vi "create demo setpoint.vi"(4 "setpoint type":T1(ring)=enum."square", 5 "manual input":dbl format="%.2f") -> (1 "setpoint":dbl(graph), 2 "show slider":bool)   [LabVIEW 2016]
doc: "This subVI creates changing set point values for the PID to track. You can choose from:\n\nsin\nsinc\natan\nsquare\ntriangle\nsawtooth\nrandom\nmanual"
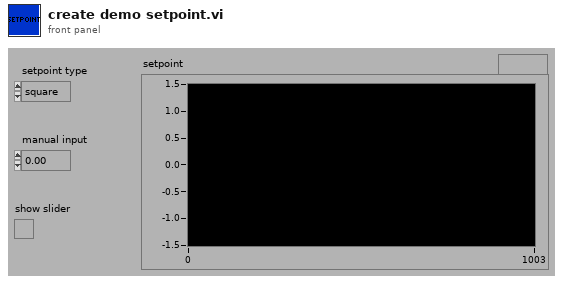
[diagram p1: front panel]
types:
  T1 = enum16{"sine", "sinc", "atan", "square", "triangle", "sawtooth", "random", "manual"}
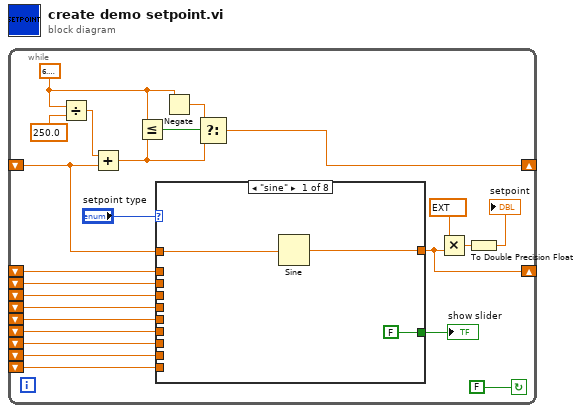
[diagram p0: block diagram]
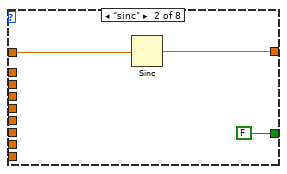
[diagram p2: hidden frame]
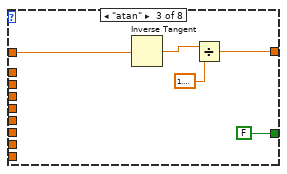
[diagram p3: hidden frame]
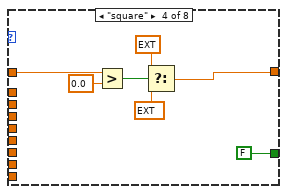
[diagram p4: hidden frame]
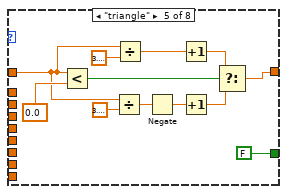
[diagram p5: hidden frame]
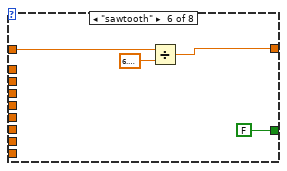
[diagram p6: hidden frame]
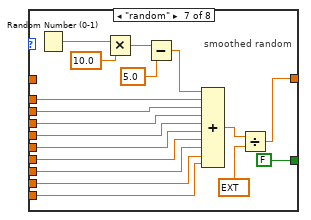
[diagram p7: hidden frame]
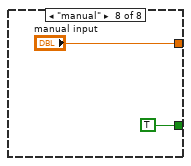
[diagram p8: hidden frame]
diagram:
  n1 = while {
    shift-left: _ -> [w8]
    shift-left: _ -> [w9]
    shift-left: _ -> [w10]
    shift-left: _ -> [w11]
    shift-left: _ -> [w13]
    shift-left: _ -> [w12]
    shift-left: _ -> [w15]
    shift-left: _ -> [w14]
    shift-left: _ -> [w16]
    shift-right: [w4] -> _
    shift-left: _ -> [w18]
    shift-right: [w17] -> _
    stop <- FALSE continue-if-true
    w7 = 6.283185307179586
    n2 = Divide(x=w7, y=250.0) -> (x/y=w22:dbl)
    n3 = Add(x=w22, y=w18) -> (x+y=w20:dbl)
    n4 = Less Or Equal?(x=w7, y=w20) -> (x <= y?=w21:bool)
    n5 = case shown="\"sine\"" "setpoint type" {
      tunnel: w18 -> [w27 w30 w35 w42 w45 w57 _ _]
      tunnel: [w26 w29 w32 w37 w44 w56 w60 "manual input"] -> w4
      tunnel: w16 -> [_ _ _ _ _ _ w71 _]
      tunnel: w15 -> [_ _ _ _ _ _ w74 _]
      tunnel: w12 -> [_ _ _ _ _ _ w73 _]
      tunnel: w14 -> [_ _ _ _ _ _ w72 _]
      tunnel: w13 -> [_ _ _ _ _ _ w65 _]
      tunnel: w11 -> [_ _ _ _ _ _ w64 _]
      tunnel: w10 -> [_ _ _ _ _ _ w63 _]
      tunnel: w9 -> [_ _ _ _ _ _ w62 _]
      tunnel: w8 -> [_ _ _ _ _ _ w61 _]
      tunnel: [FALSE ("show slider") FALSE ("show slider") FALSE ("show slider") FALSE ("show slider") FALSE ("show slider") FALSE ("show slider") FALSE ("show slider") TRUE ("show slider")] -> w6
      frame "sine" {
        n6 = Sine(x=w27) -> (sin(x)=w26:dbl)
      }
      frame "sinc" {
        n7 = Sinc(1:w30) -> (0:w29:dbl)
      }
      frame "atan" {
        n8 = Inverse Tangent(1:w35) -> (0:w34:dbl)
        n9 = Divide(x=w34, y=1.5707963267948966) -> (x/y=w32:dbl)
      }
      frame "square" {
        n10 = Greater?(x=w42, y=0.0) -> (0:w41:bool)
        n11 = Select(t=ext 1.0, s=w41, f=ext -1.0) -> (s? t:f=w37:ext)
      }
      frame "triangle" {
        n12 = Less?(x=w45, y=0.0) -> (x < y?=w53:bool)
        n13 = Divide(x=w45, y=3.141592653589793) -> (x/y=w51:dbl)
        n14 = Divide(x=w45, y=3.141592653589793) -> (x/y=w49:dbl)
        n15 = Negate(x=w51) -> (-x=w48:dbl)
        n16 = Increment(x=w49) -> (x+1=w47:dbl)
        n17 = Increment(x=w48) -> (x+1=w46:dbl)
        n18 = Select(t=w47, s=w53, f=w46) -> (s? t:f=w44:dbl)
      }
      frame "sawtooth" {
        n19 = Divide(x=w57, y=6.283185307179586) -> (x/y=w56:dbl)
      }
      frame "random" {
        # "smoothed random"
        n20 = Random Number (0-1)() -> (number: 0 to 1=w67:dbl)
        n21 = Multiply(x=w67, y=10.0) -> (x*y=w69:dbl)
        n22 = Subtract(x=w69, y=5.0) -> (x-y=w66:dbl)
        n23 = Compound Arithmetic op=ADD(w66, w71, w74, w73, w72, w65, w64, w63, w62, w61) -> (w76:ext)
        n24 = Divide(x=w76, y=ext 10.0) -> (x/y=w60:ext)
      }
      frame "manual" {
      }
    }
    "show slider" <- w6
    n25 = Negate(x=w7) -> (-x=w19:dbl)
    n26 = Select(t=w19, s=w21, f=w20) -> (s? t:f=w17:dbl)
    n27 = Multiply(x=ext 100.0 ("y"), y=w4) -> (x*y=w5:ext)
    n28 = To Double Precision Float(number=w5) -> (double precision float=→"setpoint":dbl)
  }
